vi "Create Default Hierarchy Table Rows.vi"(8 "Error in":errorcluster caption="Error in (no error)", 11 "Data":T1) -> (0 "Error out":errorcluster, 3 "OK":bool)   [LabVIEW 2018]
uses:
  TypeDef/Main - Handle Heirarchy Drag&Drop - Data.ctl
  Collect Param - Bool.vi
  <vilib>/httpClient/LabVIEWHTTPClient.lvlib
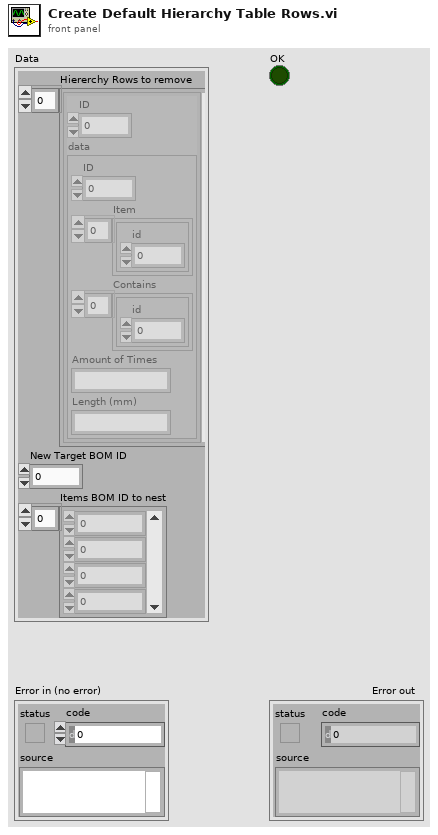
[diagram p1: front panel]
types:
  T1 = typedef "Main - Handle Heirarchy Drag&Drop - Data.ctl" = cluster{"Hiererchy Rows to remove":cluster{"ID":i32, "data":cluster{"ID":i32, "Item":cluster{"id":i32}[], "Contains":cluster{"id":i32}[], "Amount of Times":string, "Length (mm)":string}}[], "New Target BOM ID":i32, "Items BOM ID to nest":i32[]}
  T2 = typedef "LabVIEWHTTPClient.lvlib/ClientHandle.ctl" = refnum<k1>
  T3 = typedef "Param.ctl" = cluster{"Param":string, "Value":string}
  T4 = cluster{"Item":cluster{"id":i32}[], "Contains":cluster{"id":i32}[], "Amount of Times":string, "Length (mm)":string}
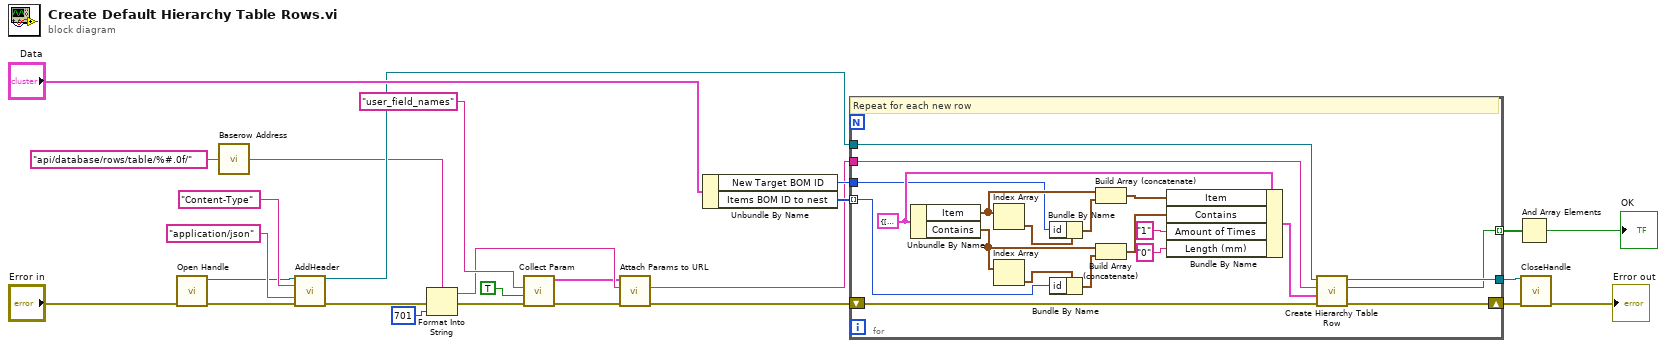
[diagram p0: block diagram]
diagram:
  n1 = call "Open Handle.vi"("error in (no error)"="Error in") -> ("error out"=w6:errorcluster, "Refnum out"=w8:T2)  [unwired: 9 in]
  n2 = call "Baserow Address.vi"("Path"="api/database/rows/table/%#.0f/" ("url")) -> ("URL + Path"=w1:string)
  n3 = call <vilib>:"AddHeader.vi"("client handle"=w8, "header"="Content-Type" ("value"), "value"="application/json", "error in (no error)"=w6) -> ("client handle out"=w7:T2, "error out"=w5:errorcluster)  [unwired: 10 in]
  n4 = Format Into String(format string=w1, error in=w5, u32 701 ("input 1")) -> (resulting string=w23:string, error out=w20:errorcluster)  [unwired: 1 in]
  n5 = call-poly "Collect Param.vi"("Error in"=w20, "Value"=TRUE, "Param Name"="user_field_names") -> ("Error out"=w21:errorcluster, "Params Array Out"=w22:T3[])  [unwired: 7 in]
  n6 = call "Attach Params to URL.vi"("Error in"=w21, "URL"=w23, "Param array"=w22) -> ("Error out"=w15:errorcluster, "URL with params"=w14:string)  [unwired: 7 in]
  n7 = Unbundle By Name("Data") -> ("New Target BOM ID"=w17:i32, "Items BOM ID to nest"=w16:i32[])
  n8 = for {
    tunnel: w17 -> [w33]
    tunnel: w16 -> [w31] mode=indexing
    shift-right: [w41] -> w12
    shift-left: w15 -> [w46]
    tunnel: w7 -> [w45]
    tunnel: w14 -> [w44]
    tunnel: [w43] -> w13
    tunnel: [w42] -> w3 mode=indexing
    w38 = T4 {"Item"=[], "Contains"=[], "Amount of Times"="", "Length (mm)"=""} ("data")
    # "Repeat for each new row"
    n9 = Unbundle By Name(w38) -> ("Item"=w37:cluster{"id":i32}[], "Contains"=w29:cluster{"id":i32}[])
    n10 = Index Array(array=w37) -> (element=w36:cluster{"id":i32})  [unwired: 1 in]
    n11 = Index Array(array=w29) -> (element=w32:cluster{"id":i32})  [unwired: 1 in]
    n12 = Bundle By Name(cluster=w36, "id"=w33) -> (w35:cluster{"id":i32})
    n13 = Bundle By Name(cluster=w32, "id"=w31) -> (w27:cluster{"id":i32})
    n14 = Build Array (concatenate)(w37, w35) -> (w34:cluster{"id":i32}[])
    n15 = Build Array (concatenate)(w29, w27) -> (w28:cluster{"id":i32}[])
    n16 = Bundle By Name(cluster=w38, "Item"=w34, "Contains"=w28, "Amount of Times"="1", "Length (mm)"="0") -> (w40:T4)
    n17 = call "Create Hierarchy Table Row.vi"("error in (no error)"=w46, "data"=w40, "URL with params"=w44, "Refnum in"=w45) -> ("error out"=w41:errorcluster, "OK"=w42:bool, "Refnum out"=w43:T2)  [unwired: 5 in]
  }
  n18 = And Array Elements(Boolean array=w3) -> (logical AND=→"OK":bool)
  n19 = call <vilib>:"CloseHandle.vi"("client handle"=w13, "error in (no error)"=w12) -> ("error out"=→"Error out":errorcluster)  [unwired: 13 in]
